vi "Setpoint Profile with Gain Scheduling on Rising and Falling.vi"() -> ()   [LabVIEW 2023]
doc: "This VI demonstrates how to specify a profile of setpoints and have the PID controller track this profile. Also this example explains how to change the PID gains when the setpoint rises or falls."
uses:
  <vilib>/addons/control/pid/pid.llb/PID (DBL).vi
  <vilib>/addons/control/pid/NI_PID_pid.lvlib
panel:
  in  "Instructions":string="Overview: This VI demonstrates how to specify a profile of setpoints and have the PID controller track this profile. Also this example explains how to change the PID gains when the setpoint rises or falls.\nInstructions:\n1. Run the VI.\n2. Verify the Setpoint Profile being generated in the Graph and notice the controller making the Process Variable track the changes.\n3. Verify that the PID Parameters Active changes from the PID Parameter on rising to the PID Parameter on falling when the profile changes direction.\n4. Verify that the profile repeats again after the last point. Click Stop to stop the VI."
  out "Falling":bool
  out "Rising":bool=TRUE
  out "Status":bool
  out "SP:":dbl(slide)=32.6797385620915 min=0.0 max=0.0 scale=0.0..100.0
  out "MV:":dbl(slide)=14.713922690048342 scale=-100.0..100.0
  out "PV:":dbl(slide)=32.905803767261574 scale=0.0..100.0
  out "PID Parameters Active":T1={"proportional gain (Kc)"=25.0, "integral time (Ti, min)"=0.02, "derivative time (Td, min)"=0.0} {"derivative time (Td, min)" format="%.3f"; "integral time (Ti, min)" format="%.3f"; "proportional gain (Kc)" format="%.3f"}
  in  "PID parameters on falling":T1={"proportional gain (Kc)"=25.0, "integral time (Ti, min)"=0.02, "derivative time (Td, min)"=0.0} {"derivative time (Td, min)" format="%.3f"; "integral time (Ti, min)" format="%.3f"; "proportional gain (Kc)" format="%.3f"}
  in  "Setpoint Profile":cluster{"time (s)":dbl, "setpoint":dbl}[](array[cluster])=[{"time (s)"=0.0, "setpoint"=0.0}, {"time (s)"=5.0, "setpoint"=40.0}, {"time (s)"=5.0, "setpoint"=80.0}, {"time (s)"=10.0, "setpoint"=80.0}, {"time (s)"=15.0, "setpoint"=0.0}] {"setpoint" format="%.2f"; "time (s)" format="%.3f"}
  in  "PID Parameter on rising":T1={"proportional gain (Kc)"=20.0, "integral time (Ti, min)"=0.01, "derivative time (Td, min)"=0.001} {"derivative time (Td, min)" format="%.3f"; "integral time (Ti, min)" format="%.3f"; "proportional gain (Kc)" format="%.3f"}
  in  "Stop":bool
  out "Graph":cluster{"initial PV":dbl, "setpoint":dbl}(graph)={"initial PV"=0.07301477741013561, "setpoint"=0.0}
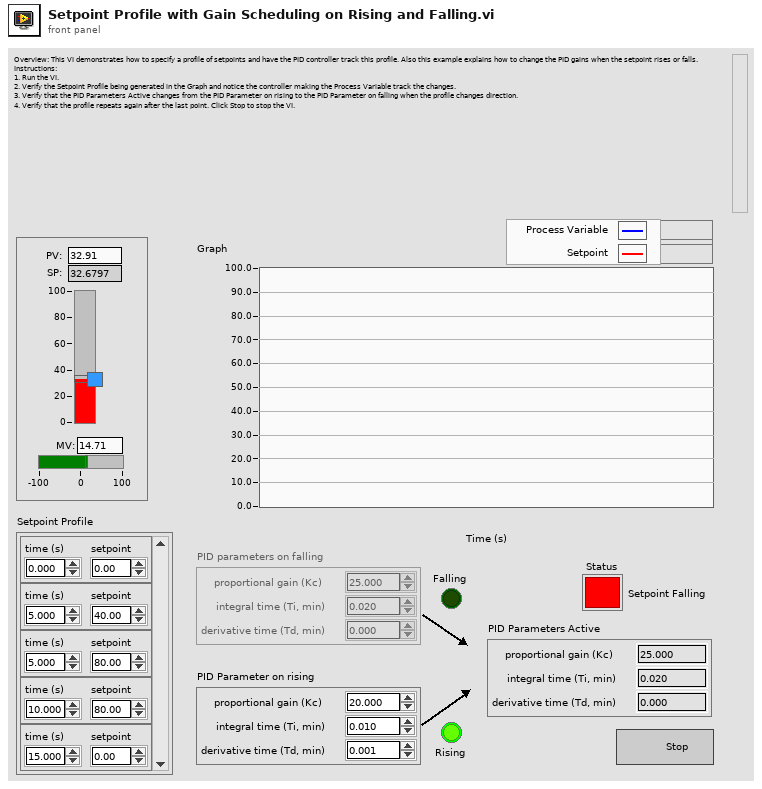
[diagram p1: front panel]
types:
  T1 = cluster{"proportional gain (Kc)":dbl, "integral time (Ti, min)":dbl, "derivative time (Td, min)":dbl}
  T2 = cluster{"static gain":dbl, "lag (min)":dbl, "dead cycles":dbl, "load %":dbl, "deadband":dbl, "noise level %":dbl, "initial PV":dbl, "initial PV 2":dbl}
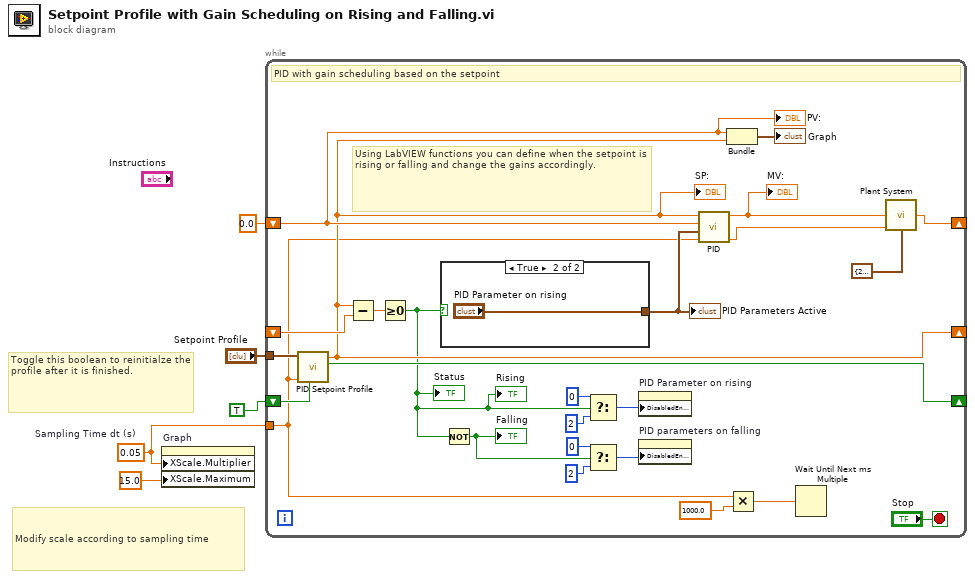
[diagram p0: block diagram]
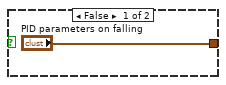
[diagram p2: hidden frame]
diagram:
  w4 = 0.05  # Sampling Time dt (s)
  # "Toggle this boolean to reinitialze the profile after it is finished."
  # "Modify scale according to sampling time"
  n1 = property on="Graph" class="WFChart (strict)"("XScale.Multiplier"=w4, "XScale.Maximum"=15.0 ("X Scale.Range:Maximum")) -> ()  [unwired: 2 in, 2 out]
  n2 = while {
    shift-left: 0.0 ("Plant Output") -> [w24]
    shift-right: [w29] -> _
    tunnel: "Setpoint Profile" -> [w27]
    tunnel: w4 -> [w7]
    shift-right: [w23] -> _
    shift-left: _ -> [w25]
    shift-right: [w20] -> _
    shift-left: TRUE ("profile complete?") -> [w19]
    stop <- "Stop" stop-if-true
    # "Using LabVIEW functions you can define when the setpoint is rising or falling and change the gains accordingly."
    # "PID with gain scheduling based on the setpoint"
    n3 = call <vilib>:"PID Setpoint Profile.vi"("reinitialize? (F)"=w19, "dt (s)"=w7, "setpoint profile"=w27) -> ("profile complete?"=w20:bool, "setpoint"=w23:dbl)  [unwired: 3 in, 2 out]
    "SP:" <- w23
    n4 = Subtract(x=w23, y=w25) -> (x-y=w26:dbl)
    n5 = Greater Or Equal To 0?(x=w26) -> (x >= 0?=w17:bool)
    "Status" <- w17
    "Rising" <- w17
    n6 = case shown="True" w17 {
      tunnel: ["PID parameters on falling" "PID Parameter on rising"] -> w28
      frame False {
      }
      frame True {
      }
    }
    "PID Parameters Active" <- w28
    n7 = Not(x=w17) -> (.not. x?=w11:bool)
    "Falling" <- w11
    n8 = Select(t=0, s=w17, f=2) -> (s? t:f=w16:i32)
    n9 = Select(t=0, s=w11, f=2) -> (s? t:f=w10:i32)
    n10 = property on="PID Parameter on rising" class="Clust (strict)"("DisabledEnum"=w16) -> ()  [unwired: 2 in, 2 out]
    n11 = property on="PID parameters on falling" class="Clust (strict)"("DisabledEnum"=w10) -> ()  [unwired: 2 in, 2 out]
    n12 = call-poly <vilib>:"PID.vi"("dt (s)"=w7, "PID gains"=w28, "process variable"=w24, "setpoint"=w23) -> ("dt out (s)"=w6:dbl, "output"=w21:dbl)  [unwired: 6 in]
    "MV:" <- w21
    n13 = Bundle("Plant Output"=w24, "setpoint"=w23) -> (→"Graph":cluster{"Plant Output":dbl, "setpoint":dbl})  [unwired: 1 in]
    n14 = Multiply(x=w7, y=1000.0) -> (x*y=w9:dbl)
    n15 = Wait Until Next ms Multiple(millisecond multiple=w9) -> ()  [unwired: 1 out]
    n16 = call "Plant System.vi"("Plant Input"=w21, "dt (s)"=w6, "process parameters"=T2 {"static gain"=2.5, "lag (min)"=6.0, "dead cycles"=0.1, "load %"=40.0, "deadband"=2.0, "noise level %"=0.25, "initial PV"=0.0, "initial PV 2"=0.0}) -> ("Plant Output"=w29:dbl)  [unwired: 12 in]
    "PV:" <- w24
  }
